vi "Check wavelengths value.vi"(3 "LowerCalibrationWl":dbl, 4 "UpperCalibrationWl":dbl, 5 "wavelength_nm":dbl) -> (0 "LowerCalibrationWl out":dbl, 1 "UpperCalibrationWl out":dbl, 2 "wavelength_nm out":dbl)   [LabVIEW 2020]
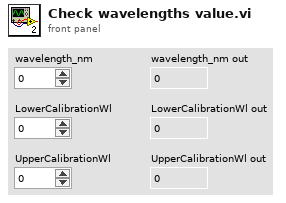
[diagram p1: front panel]
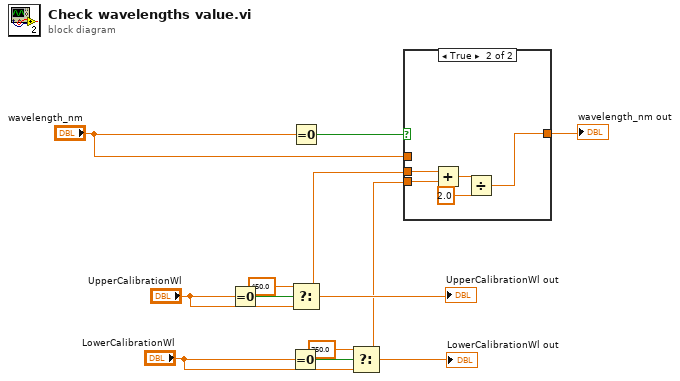
[diagram p0: block diagram]
diagram:
  n1 = Equal To 0?(x="UpperCalibrationWl") -> (x = 0?=w11:bool)
  n2 = Equal To 0?(x="LowerCalibrationWl") -> (x = 0?=w9:bool)
  n3 = Equal To 0?(x="wavelength_nm") -> (x = 0?=w3:bool)
  n4 = Select(t=450.0, s=w11, f="UpperCalibrationWl") -> (s? t:f=w2:dbl)
  "UpperCalibrationWl out" <- w2
  n5 = Select(t=750.0, s=w9, f="LowerCalibrationWl") -> (s? t:f=w1:dbl)
  "LowerCalibrationWl out" <- w1
  n6 = case shown="True" w3 {
    tunnel: "wavelength_nm" -> [w12 _]
    tunnel: w2 -> [_ w17]
    tunnel: w1 -> [_ w16]
    tunnel: [w12 w13] -> w4
    frame False {
    }
    frame True {
      n7 = Add(x=w17, y=w16) -> (x+y=w15:dbl)
      n8 = Divide(x=w15, y=2.0) -> (x/y=w13:dbl)
    }
  }
  "wavelength_nm out" <- w4
